vi "AllThings.vi"   [LabVIEW 2024]
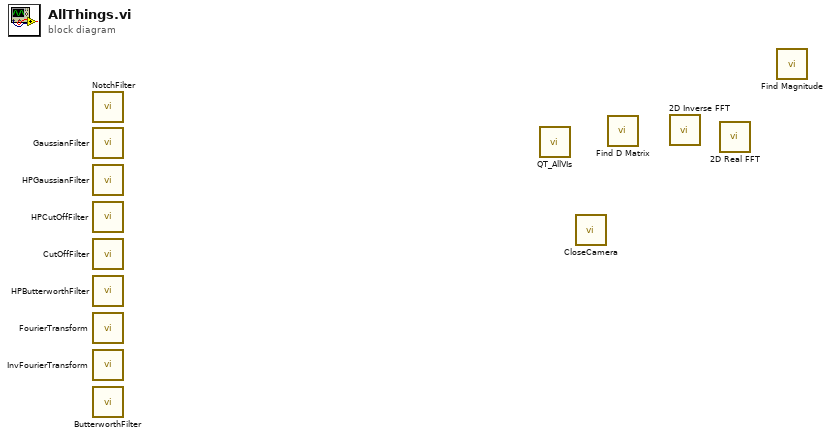
[diagram p0: block diagram]
diagram:
  n1 = call <userlib>:"NotchFilter.vi"() -> ()  [unwired: 2 in, 2 out]
  n2 = call <userlib>:"GaussianFilter.vi"() -> ()  [unwired: 3 in, 2 out]
  n3 = call <userlib>:"HPGaussianFilter.vi"() -> ()  [unwired: 2 in, 2 out]
  n4 = call <userlib>:"HPCutOffFilter.vi"() -> ()  [unwired: 2 in, 2 out]
  n5 = call <userlib>:"CutOffFilter.vi"() -> ()  [unwired: 2 in, 2 out]
  n6 = call <userlib>:"HPButterworthFilter.vi"() -> ()  [unwired: 3 in, 2 out]
  n7 = call <userlib>:"FourierTransform.vi"() -> ()  [unwired: 2 in, 2 out]
  n8 = call <userlib>:"InvFourierTransform.vi"() -> ()  [unwired: 3 in, 1 out]
  n9 = call <userlib>:"ButterworthFilter.vi"() -> ()  [unwired: 3 in, 2 out]
  n10 = call <userlib>:"QT_AllVIs.vi"() -> ()  [unwired: 1 in]
  n11 = call <userlib>:"CloseCamera.vi"() -> ()  [unwired: 3 in, 1 out]
  n12 = call <userlib>:"Find D Matrix.vi"() -> ()  [unwired: 1 in, 1 out]
  n13 = call <userlib>:"2D Inverse FFT.vi"() -> ()  [unwired: 1 in, 1 out]
  n14 = call <userlib>:"2D Real FFT.vi"() -> ()  [unwired: 1 in, 1 out]
  n15 = call <userlib>:"Find Magnitude.vi"() -> ()  [unwired: 1 in, 1 out]
